vi "URL Read 3.vi"(4 "error in (no error)":errorcluster, 6 "Container State":T2, 7 "Display State In":T1) -> (0 "error out":errorcluster, 2 "Value":string, 3 "Display State Out":T1)   [LabVIEW 2020, in "WebView2 XControl.lvlib" / "WebView2 Control.xctl"]
uses:
  WebView2 Control.xctl
  <vilib>/_xctls/Container State.ctl
  State.ctl
  Webview2 Lib/WebView2 Control Object/WebView2 Control.lvclass
  Webview2 Lib/WebView2 Control Object/Read URL.vi
  <vilib>/_xctls/XControlSupport.lvlib
panel:
  # "Replace the Value Indicator below with an Indicator of desired type.\nDo not remove this Indicator or the others from the connector pane. \nDo not change the connector pane pattern.\nThe Value Indicator should always be the second terminal from top on the output side in the connector pane."
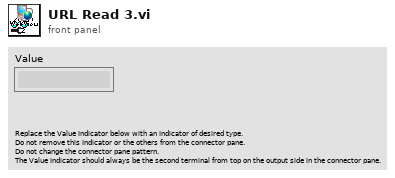
[diagram p1: front panel]
types:
  T1 = typedef "WebView2 XControl.lvlib/WebView2 Control.xctl/State.ctl" = cluster{"Control Object Ref":refnum<data-value>}
  T2 = typedef "XControlSupport.lvlib/Container State.ctl" = cluster{"Indicator?":bool, "Run Mode?":bool, " Refnum":refnum<vi>}
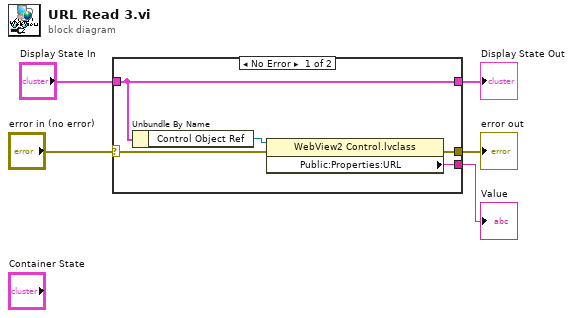
[diagram p0: block diagram]
diagram:
  n1 = case shown="No Error" "error in (no error)" {
    selector: "error in (no error)" -> [w7 w12]
    tunnel: [w10 w12] -> w3
    tunnel: [w9 _] -> w5
    tunnel: "Display State In" -> [w6 w11]
    tunnel: [w6 w11] -> w1
    frame No Error {
      n2 = Unbundle By Name(w6) -> ("Control Object Ref"=w8:refnum<data-value>)
      n3 = property class="WebView2 Control.lvclass"(reference=w8, error in=w7) -> (error out=w10:errorcluster, "Public:Properties:URL"=w9:string)  [unwired: 1 out]
    }
    frame Error {
    }
  }
  "error out" <- w3
  "Display State Out" <- w1
  "Value" <- w5
